vi "Read State.vi"(8 "error in (no error)":errorcluster, 11 "Change Speaker State in":refnum<class "Change Speaker State.lvclass">) -> (0 "error out":errorcluster, 2 "State":bool, 3 "Change Speaker State out":refnum<class "Change Speaker State.lvclass">)   [LabVIEW 2014, in "ePAS Library.lvlib" / "Change Speaker State.lvclass"]
uses:
  Change Speaker State.lvclass
  Change Speaker State.lvclass/Change Speaker State.ctl
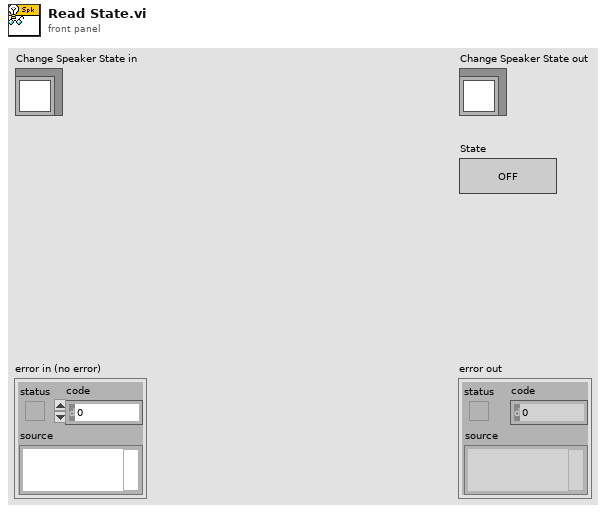
[diagram p1: front panel]
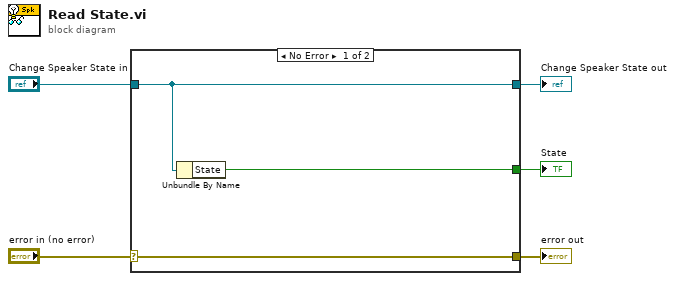
[diagram p0: block diagram]
diagram:
  n1 = case shown="No Error" "error in (no error)" {
    selector: "error in (no error)" -> [w8 w9]
    tunnel: [w8 w9] -> w4
    tunnel: [w7 w10] -> w2
    tunnel: "Change Speaker State in" -> [w7 w10]
    tunnel: [w6 _] -> w1
    frame No Error {
      n2 = Unbundle By Name(w7) -> ("State"=w6:bool)
    }
    frame Error {
    }
  }
  "error out" <- w4
  "Change Speaker State out" <- w2
  "State" <- w1
